vi "Get Connection Status.vi"(8 "error in (no error)":errorcluster) -> (0 "error out":errorcluster, 3 "connected":bool)   [LabVIEW 2021, in "AudioGenManageConnectionProcess.lvlib"]
uses:
  AudioGenManageConnectionProcess.lvlib
  <vilib>/addons/PointValueMap/subVIs/Point_Read_variant.vi
  <vilib>/addons/PointValueMap/PointValueMap.lvlib
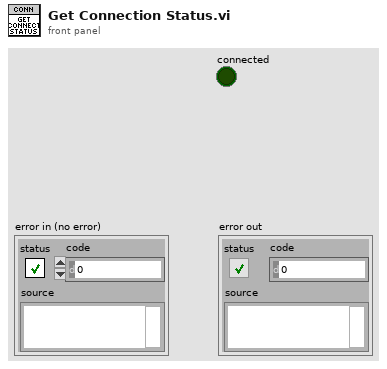
[diagram p1: front panel]
types:
  T1 = typedef "PointValueMap.lvlib/PointMap.ctl" = refnum<data-value>
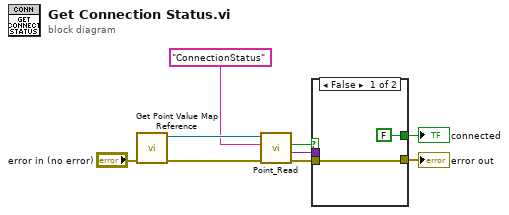
[diagram p0: block diagram]
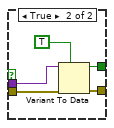
[diagram p2: hidden frame]
diagram:
  n1 = call "Get Point Value Map Reference.vi"("error in (no error)"="error in (no error)") -> ("error out"=w7:errorcluster, "Map Out"=w8:T1)  [unwired: 9 in]
  n2 = call-poly <vilib>:"Point_Read.vi"("Error In"=w7, "Tag"="ConnectionStatus", "Map"=w8) -> ("Error Out"=w5:errorcluster, "Value"=w3:variant, "Found?"=w1:bool)  [unwired: 3 in, 3 out]
  n3 = case shown="False" w1 {
    tunnel: w5 -> [w11 w16]
    tunnel: [w11 w15] -> w4
    tunnel: w3 -> [_ w14]
    tunnel: [FALSE w12] -> w2
    frame False {
    }
    frame True {
      n4 = Variant To Data(error in=w16, type=TRUE, Variant=w14) -> (data=w12:bool, error out=w15:errorcluster)
    }
  }
  "error out" <- w4
  "connected" <- w2
